vi "UpdateS4GUI_JSON_string.vi"(8 "error in (no error)":errorcluster, 10 "status":string, 11 "Interface in":refnum<class "Interface.lvclass">) -> (0 "error out":errorcluster, 2 "S4GUI JSON string rx":T1={"OBSERVER"="", "OBJECT"="", "CTRLINTE"="S4GUI", "PROJID"="", "SYNCMODE"="SYNC", "INSTMODE"="PHOT", "FILTER"="CLEAR", "OBSTYPE"="", "CHANNEL 1"=FALSE, "CHANNEL 2"=FALSE, "CHANNEL 3"=FALSE, "CHANNEL 4"=FALSE, "TCSMODE"=FALSE, "COMMENT"="", "broker"="S4GUI", "GUIVRSN"="", "timestamp"="S4GUI"}, 3 "Interface out":refnum<class "Interface.lvclass">)   [LabVIEW 2018, in "Interface.lvclass"]
uses:
  Interface.lvclass
panel:
  in  "S4GUI JSON string":T1={"OBSERVER"="", "OBJECT"="", "CTRLINTE"="S4GUI", "PROJID"="", "SYNCMODE"="SYNC", "INSTMODE"="PHOT", "FILTER"="CLEAR", "OBSTYPE"="", "CHANNEL 1"=FALSE, "CHANNEL 2"=FALSE, "CHANNEL 3"=FALSE, "CHANNEL 4"=FALSE, "TCSMODE"=FALSE, "COMMENT"="", "broker"="S4GUI", "GUIVRSN"="", "timestamp"="S4GUI"}
  in  "Cluster S4GUI JSON":cluster{"S4GUI JSON string":string}
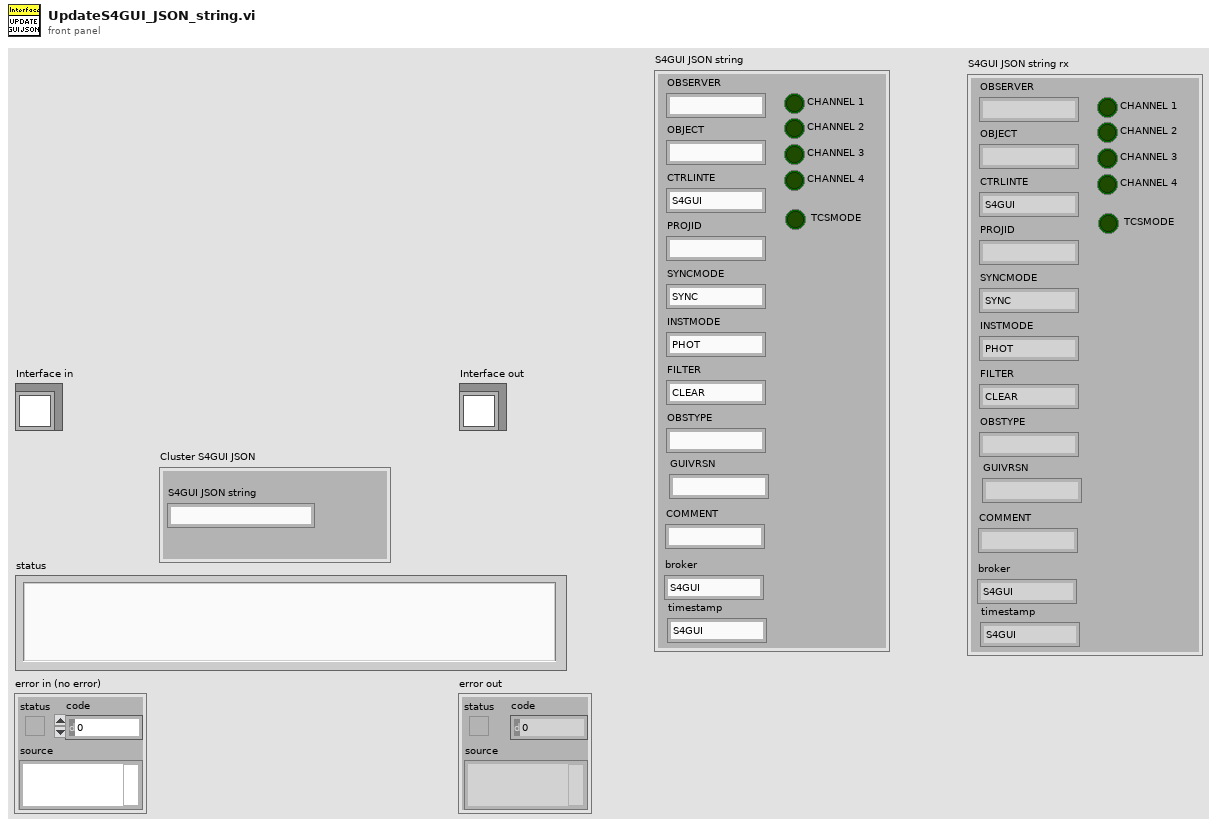
[diagram p1: front panel]
types:
  T1 = cluster{"OBSERVER":string, "OBJECT":string, "CTRLINTE":string, "PROJID":string, "SYNCMODE":string, "INSTMODE":string, "FILTER":string, "OBSTYPE":string, "CHANNEL 1":bool, "CHANNEL 2":bool, "CHANNEL 3":bool, "CHANNEL 4":bool, "TCSMODE":bool, "COMMENT":string, "broker":string, "GUIVRSN":string, "timestamp":string}
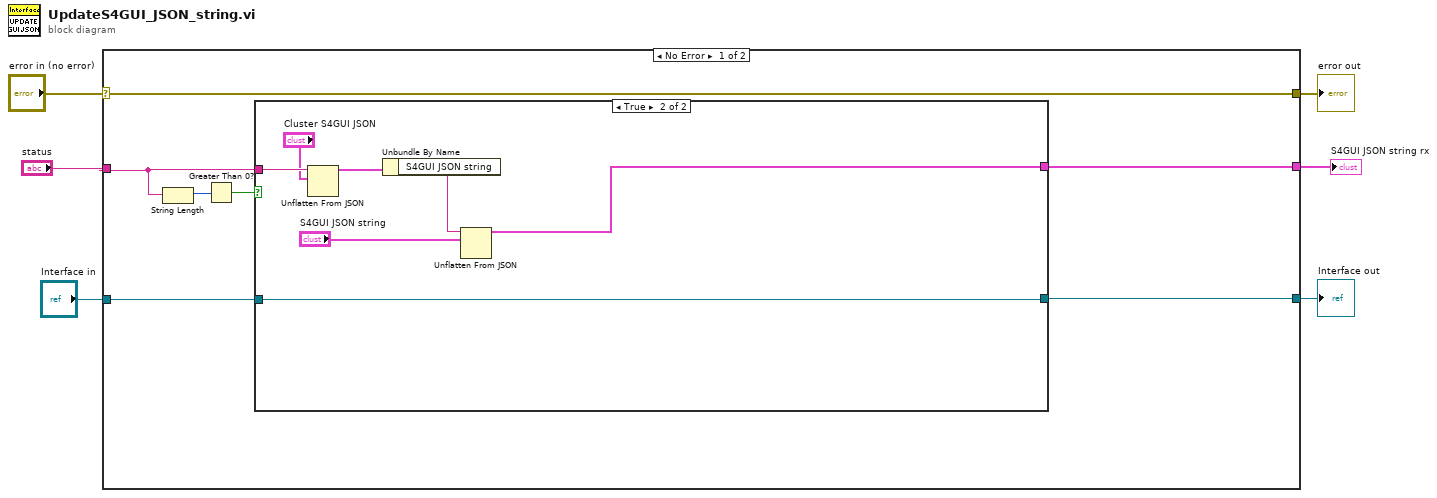
[diagram p0: block diagram]
diagram:
  n1 = case shown="No Error" "error in (no error)" {
    selector: "error in (no error)" -> [w13 w23]
    tunnel: [w13 w23] -> w5
    tunnel: [w12 w22] -> w3
    tunnel: "Interface in" -> [w10 w22]
    tunnel: "status" -> [w8 _]
    tunnel: [w7 _] -> w1
    frame No Error {
      n2 = String Length(string=w8) -> (length=w11:i32)
      n3 = Greater Than 0?(x=w11) -> (x > 0?=w9:bool)
      n4 = case shown="True" w9 {
        tunnel: [w14 w16] -> w12
        tunnel: w8 -> [_ w21]
        tunnel: w10 -> [w14 w16]
        tunnel: [_ w17] -> w7
        frame False {
        }
        frame True {
          n5 = Unflatten From JSON(JSON string=w21, type and defaults="Cluster S4GUI JSON") -> (value=w19:cluster{"S4GUI JSON string":string})  [unwired: 5 in, 1 out]
          n6 = Unbundle By Name(w19) -> ("S4GUI JSON string"=w18:string)
          n7 = Unflatten From JSON(JSON string=w18, type and defaults="S4GUI JSON string") -> (value=w17:T1)  [unwired: 5 in, 1 out]
        }
      }
    }
    frame Error {
    }
  }
  "error out" <- w5
  "Interface out" <- w3
  "S4GUI JSON string rx" <- w1
